vi "Get_Address_Device.vi"(8 "error in (no error)":errorcluster caption="entrée d'erreur (pas d'erreur)", 11 "Class Relay_Board (Default) en entrée":refnum<class "Class Relay_Board (Default).lvclass">) -> (0 "error out":errorcluster caption="sortie d'erreur", 2 "Device COM":string, 3 "Class Relay_Board (Default) en sortie":refnum<class "Class Relay_Board (Default).lvclass">)   [LabVIEW 2020, in "Library Instrument & Equipement.lvlib" / "Library Relay_Board.lvlib" / "Class Relay_Board (Default).lvclass"]
uses:
  Class Relay_Board (Default).lvclass
  Class Relay_Board (Default).lvclass/Class Relay_Board (Default).ctl
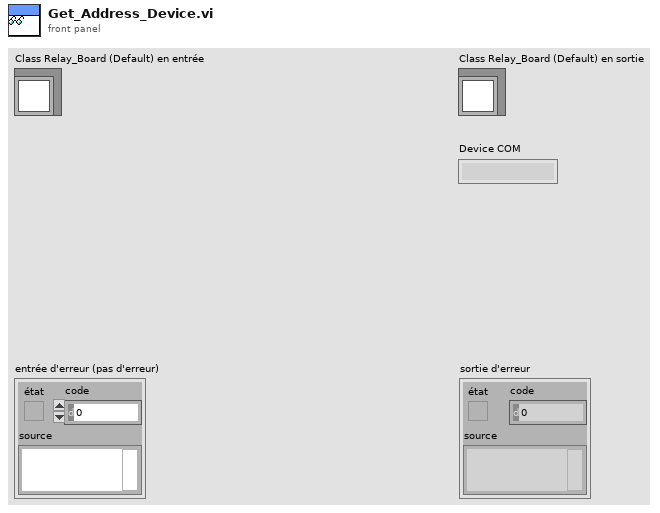
[diagram p1: front panel]
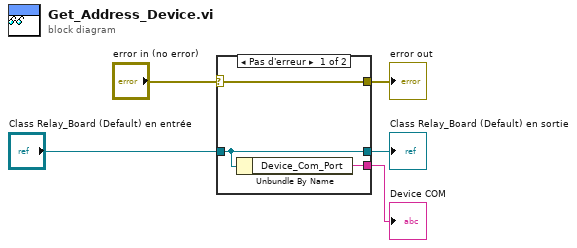
[diagram p0: block diagram]
diagram:
  n1 = case shown="Pas d'erreur" "error in (no error)" {
    selector: "error in (no error)" -> [w8 w9]
    tunnel: [w8 w9] -> w4
    tunnel: [w7 w10] -> w2
    tunnel: "Class Relay_Board (Default) en entrée" -> [w7 w10]
    tunnel: [w6 _] -> w1
    frame No Error {
      n2 = Unbundle By Name(w7) -> ("Device_Com_Port"=w6:string)
    }
    frame Error {
    }
  }
  "error out" <- w4
  "Class Relay_Board (Default) en sortie" <- w2
  "Device COM" <- w1
